vi "FTW-ScripterStep-Base_ReportResults.vi"(0 "FTW-ScripterStep-Base In":refnum<class "FTW-ScripterStep-Base.lvclass">, 5 "Passed":bool, 7 "Additional Results":variant, 11 "error in (no error)":errorcluster) -> (4 "FTW-ScripterStep-Base Out":refnum<class "FTW-ScripterStep-Base.lvclass">, 15 "error out":errorcluster)   [LabVIEW 2015, in "FTW-ScripterStep-Base.lvclass"]
uses:
  FTW-ScripterStep-Base.lvclass
  source/actor/Connector/FTW-ActorConnector.lvclass
  Scripter/FTW-Scripter-Results.ctl
  source/container/FTW-Container.lvclass
  FTW-ScripterStep-Base.lvclass/FTW-ScripterStep-Base.ctl
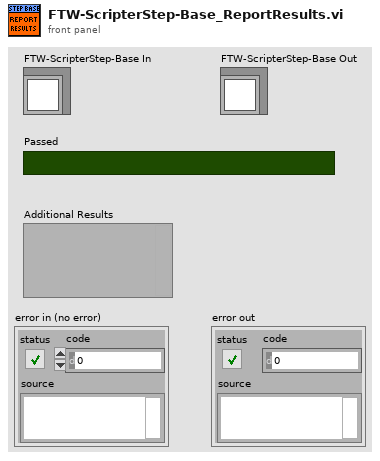
[diagram p1: front panel]
types:
  T1 = typedef "FTW-Scripter-Results.ctl" = cluster{"Start Time":timestamp, "Elapsed Time":dbl, "Passed":bool, "Additional Results":refnum<class "FTW-Container.lvclass">}
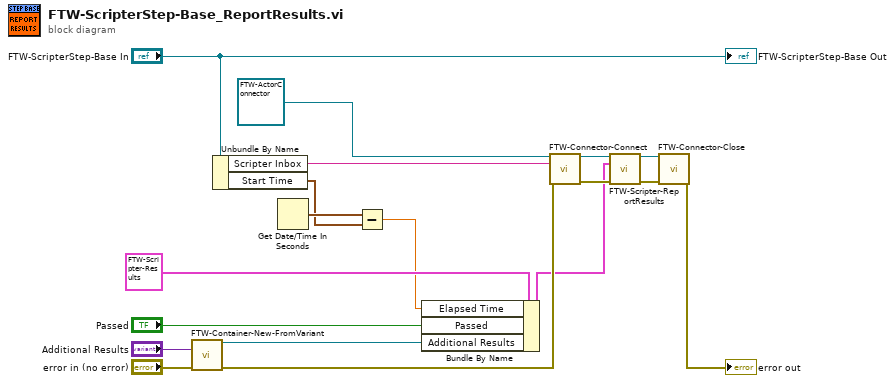
[diagram p0: block diagram]
diagram:
  n1 = call "FTW-Container-New-FromVariant.vi"("Variant"="Additional Results", "error in"="error in (no error)") -> ("FTW-Container"=w8:refnum<class "FTW-Container.lvclass">, "error out"=w10:errorcluster)  [unwired: 12 in]
  n2 = Unbundle By Name("FTW-ScripterStep-Base In") -> ("Scripter Inbox"=w4:string, "Start Time"=w2:timestamp)
  n3 = Get Date/Time In Seconds() -> (seconds since 1Jan1904=w3:timestamp)
  n4 = Subtract(x=w3, y=w2) -> (x-y=w1:dbl)
  n5 = Bundle By Name(cluster=T1 {"Start Time"=timestamp(0 s since 1904-01-01), "Elapsed Time"=0.0, "Passed"=FALSE, "Additional Results"=refnum} ("Results"), "Elapsed Time"=w1, "Passed"="Passed", "Additional Results"=w8) -> (w7:T1)
  n6 = call-dynamic "FTW-Connector-Connect.vi"("FTW Actor Connector Type"=refnum<class "FTW-ActorConnector.lvclass"> refnum, "Instance Inbox Address"=w4, "error in"=w10) -> ("FTW Actor Connector"=w17:refnum<class "FTW-ActorConnector.lvclass">, "error out"=w13:errorcluster)  [unwired: 11 in]
  n7 = call "FTW-Scripter-ReportResults.vi"("FTW Actor Connector In"=w17, "Results"=w7, "error in (no error)"=w13) -> ("FTW Actor Connector"=w18:refnum<class "FTW-ActorConnector.lvclass">, "error out"=w16:errorcluster)  [unwired: 9 in, 2 out]
  n8 = call-dynamic "FTW-Connector-Close.vi"("FTW Actor Connector"=w18, "error in"=w16) -> ("error out"=→"error out":errorcluster)  [unwired: 13 in]
  "FTW-ScripterStep-Base Out" <- "FTW-ScripterStep-Base In"
